vi "Day04-1.vi"() -> ()   [LabVIEW 2021]
uses:
  <vilib>/Utility/error.llb/whitespace.ctl
panel:
  out "Array 2":i32[][][](array[numeric])
  out "Array":i32[][](array[numeric])
  out "Answer":i32
  out "Bingo Numbers":string[](array[string])
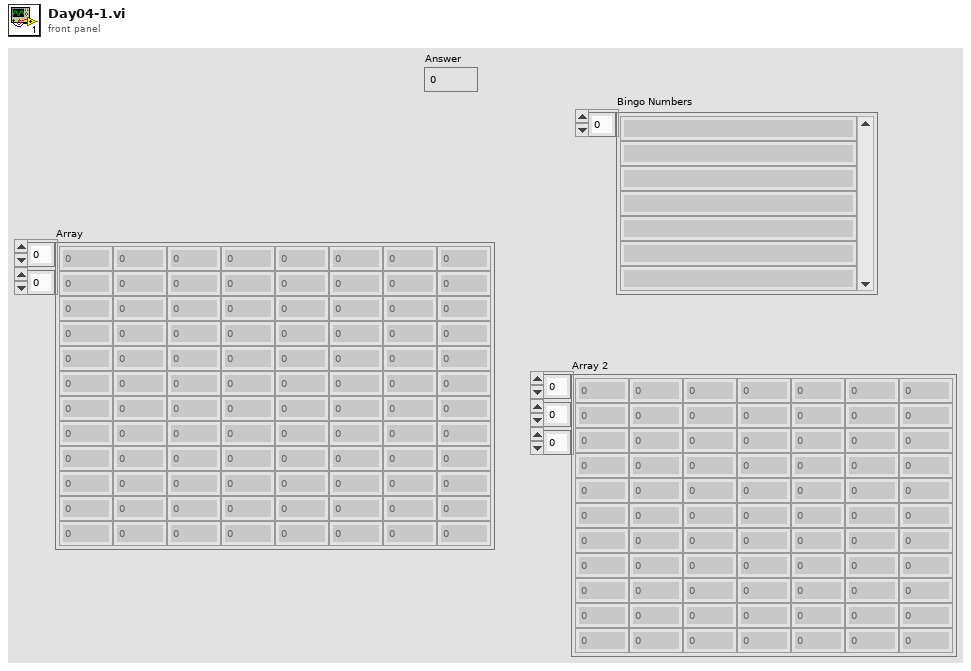
[diagram p1: front panel]
types:
  T1 = typedef "whitespace.ctl" = u16
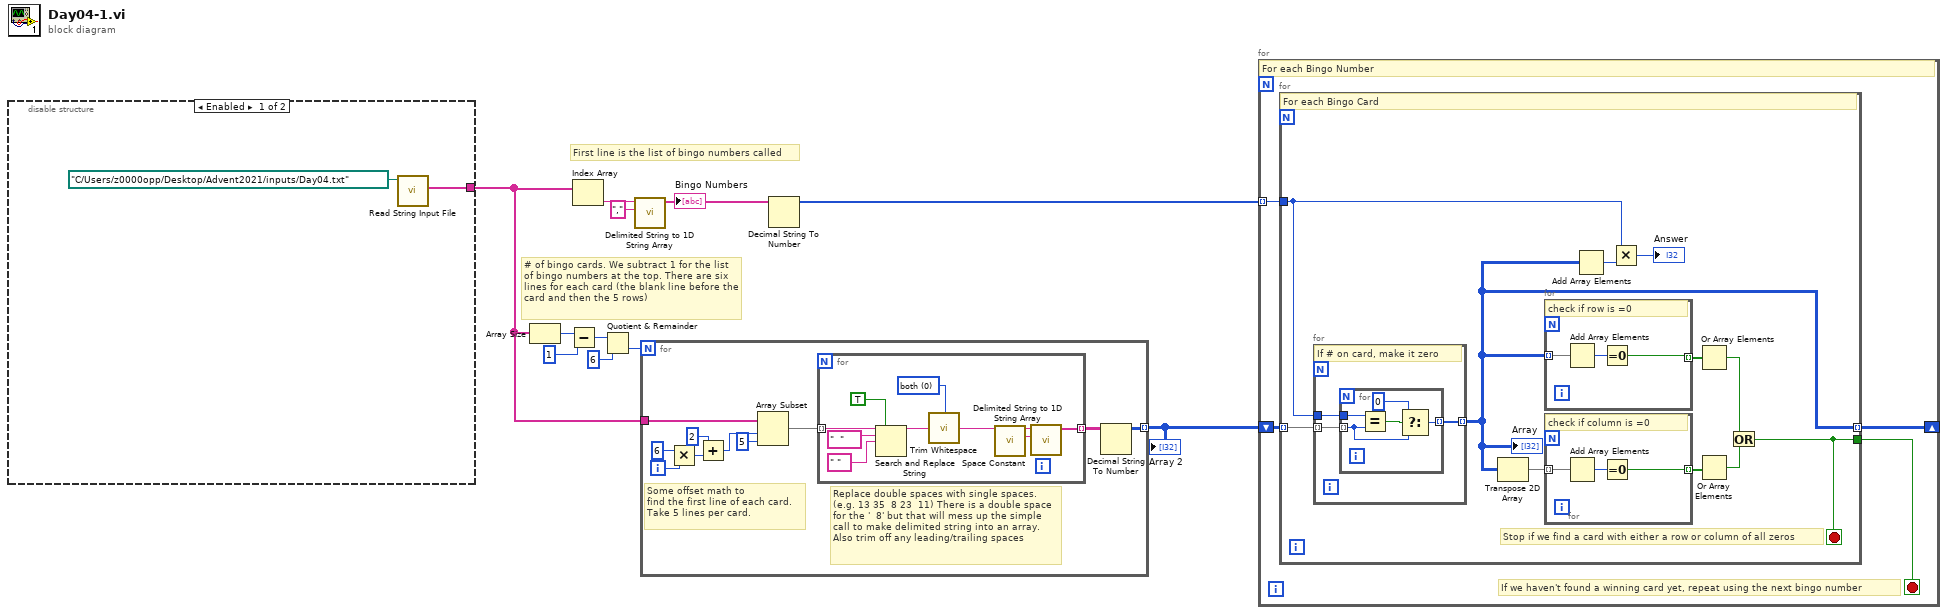
[diagram p0: block diagram]
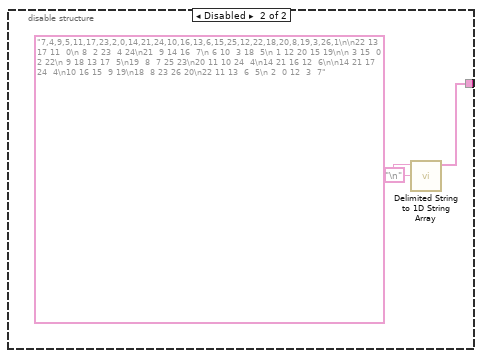
[diagram p2: hidden frame]
diagram:
  # "# of bingo cards. We subtract 1 for the list of bingo numbers at the top. There are six lines for each card (the blank line before the card and then the 5 rows)"
  # "First line is the list of bingo numbers called"
  n1 = disable-structure shown="Enabled" {
    disable-tunnel: [w12 w14] -> w9
    frame Enabled {
      n2 = call "Read String Input File.vi"("file path (dialog if empty)"=path "C:/Users/z0000opp/Desktop/Advent2021/inputs/Day04.txt") -> ("input values"=w12:string[])  [unwired: 10 in]
    }
    frame Disabled {
      n3 = call <vilib>:"Delimited String to 1D String Array.vi"("delimiter"="\n", "delimited string"="7,4,9,5,11,17,23,2,0,14,21,24,10,16,13,6,15,25,12,22,18,20,8,19,3,26,1\n\n22 13 17 11  0\n 8  2 23  4 24\n21  9 14 16  7\n 6 10  3 18  5\n 1 12 20 15 19\n\n 3 15  0  2 22\n 9 18 13 17  5\n19  8  7 25 23\n20 11 10 24  4\n14 21 16 12  6\n\n14 21 17 24  4\n10 16 15  9 19\n18  8 23 26 20\n22 11 13  6  5\n 2  0 12  3  7") -> ("string array"=w14:string[])  [unwired: 9 in]
    }
  }
  n4 = Array Size(array=w9) -> (size(s)=w8:i32)
  n5 = Subtract(x=w8, y=1) -> (x-y=w6:i32)
  n6 = Index Array(array=w9) -> (element=w11:string)  [unwired: 1 in]
  n7 = Quotient & Remainder(x=w6, y=6) -> (floor(x/y)=w4:i32)  [unwired: 1 out]
  n8 = call <vilib>:"Delimited String to 1D String Array.vi"("delimiter"=",", "delimited string"=w11) -> ("string array"=w3:string[])  [unwired: 9 in]
  "Bingo Numbers" <- w3
  n9 = for {
    N: w4 -> [_]
    tunnel: w9 -> [w26]
    tunnel: [w17] -> w2 mode=indexing
    i -> [w25]
    # "Replace double spaces with single spaces.\n(e.g. 13 35  8 23  11) There is a double space\nfor the '  8' but that will mess up the simple\ncall to make delimited string into an array.\nAlso trim off any leading/trailing spaces"
    # "Some offset math to\nfind the first line of each card.\nTake 5 lines per card."
    n10 = Multiply(x=6, y=w25) -> (x*y=w23:i32)
    n11 = Add(x=2, y=w23) -> (x+y=w21:i32)
    n12 = Array Subset(array=w26, index=w21, length=5) -> (w20:string[])
    n13 = for {
      tunnel: w20 -> [w34] mode=indexing
      tunnel: [w35] -> w18 mode=indexing
      w27 = T1 0 items=["both", "start of string", "end of string"] ("location (both)")
      n14 = Search and Replace String(replace all?=TRUE ("replace all? (F)"), input string=w34, search string="  ", replace string=" ") -> (result string=w30:string)  [unwired: 4 in, 3 out]
      n15 = call <vilib>:"Trim Whitespace.vi"("string"=w30, "location (both)"=w27) -> ("trimmed string"=w28:string)
      n16 = call <vilib>:"Space Constant.vi"() -> ("String"=w29:string)
      n17 = call <vilib>:"Delimited String to 1D String Array.vi"("delimiter"=w29, "delimited string"=w28) -> ("string array"=w35:string[])  [unwired: 9 in]
    }
    n18 = Decimal String To Number(string=w18) -> (number=w17:i32[][])  [unwired: 2 in, 1 out]
  }
  "Array 2" <- w2
  n19 = Decimal String To Number(string=w3) -> (number=w1:i32[])  [unwired: 2 in, 1 out]
  n20 = for {
    tunnel: w1 -> [w38] mode=indexing
    shift-right: [w36] -> _
    shift-left: w2 -> [w39]
    stop <- w37 stop-if-true
    # "If we haven't found a winning card yet, repeat using the next bingo number"
    # "For each Bingo Number"
    n21 = for {
      tunnel: w39 -> [w50] mode=indexing
      tunnel: w38 -> [w43]
      tunnel: [w41] -> w37
      tunnel: [w40] -> w36 mode=indexing
      stop <- w41 stop-if-true
      # "Stop if we find a card with either a row or column of all zeros"
      # "For each Bingo Card"
      n22 = for {
        tunnel: w50 -> [w59] mode=indexing
        tunnel: w43 -> [w58]
        tunnel: [w57] -> w40 mode=indexing
        # "If # on card, make it zero"
        n23 = for {
          tunnel: w59 -> [w62] mode=indexing
          tunnel: w58 -> [w64]
          tunnel: [w61] -> w57 mode=indexing
          n24 = Equal?(x=w64, y=w62) -> (x = y?=w63:bool)
          n25 = Select(t=0, s=w63, f=w62) -> (s? t:f=w61:i32)
        }
      }
      "Array" <- w40
      n26 = Transpose 2D Array(2D array=w40) -> (transposed array=w49:i32[][])
      n27 = for {
        tunnel: w40 -> [w56] mode=indexing
        tunnel: [w54] -> w48 mode=indexing
        # "check if row is =0"
        n28 = Add Array Elements(numeric array=w56) -> (sum=w55:i32)
        n29 = Equal To 0?(x=w55) -> (x = 0?=w54:bool)
      }
      n30 = for {
        tunnel: w49 -> [w53] mode=indexing
        tunnel: [w51] -> w47 mode=indexing
        # "check if column is =0"
        n31 = Add Array Elements(numeric array=w53) -> (sum=w52:i32)
        n32 = Equal To 0?(x=w52) -> (x = 0?=w51:bool)
      }
      n33 = Add Array Elements(numeric array=w40) -> (sum=w44:i32)
      n34 = Multiply(x=w43, y=w44) -> (x*y=→"Answer":i32)
      n35 = Or Array Elements(Boolean array=w48) -> (logical OR=w45:bool)
      n36 = Or Array Elements(Boolean array=w47) -> (logical OR=w46:bool)
      n37 = Or(x=w45, y=w46) -> (x .or. y?=w41:bool)
    }
  }
